vi "Istwerte eintragen.vi"(9 "Auswahlfelder":T1) -> (1 "Aktuelle Werte":T3 {"Zahlen-Ausgabefeld 16" format="%#.2f"; "Zahlen-Ausgabefeld 15" format="%#.2f"; "Zahlen-Ausgabefeld 14" format="%#.2f"; "Zahlen-Ausgabefeld 13" format="%#.2f"; "Zahlen-Ausgabefeld 12" format="%#.2f"; "Zahlen-Ausgabefeld 11" format="%#.2f"; "Zahlen-Ausgabefeld 10" format="%#.2f"; "Zahlen-Ausgabefeld 9" format="%#.2f"; "Zahlen-Ausgabefeld 8" format="%#.2f"; "Zahlen-Ausgabefeld 7" format="%#.2f"; "Zahlen-Ausgabefeld 6" format="%#.2f"; "Zahlen-Ausgabefeld 5" format="%#.2f"; "Zahlen-Ausgabefeld 4" format="%#.2f"; "Zahlen-Ausgabefeld 3" format="%#.2f"; "Zahlen-Ausgabefeld 2" format="%#.2f"; "Zahlen-Ausgabefeld" format="%#.2f"})   [LabVIEW 2020, in "Gaszuordnung AO.lvlib"]
uses:
  Gaszuordnung AO.lvlib
  Aktuelle Werte Anzeige.ctl
  Auswahlfelder Anzeige.ctl
  Visualisierungs Elemente/Auswahlfeld.ctl
  Messdaten/Messdaten.lvlib
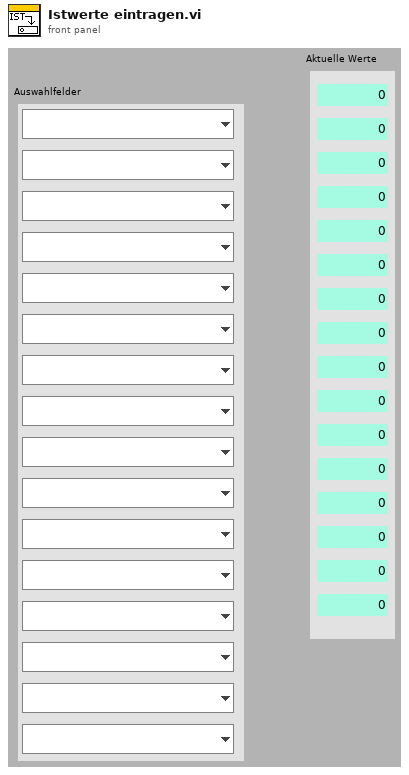
[diagram p1: front panel]
types:
  T1 = typedef "Gaszuordnung AO.lvlib/Auswahlfelder Anzeige.ctl" = cluster{"Auswahl":T2, "Auswahl 2":T2, "Auswahl 3":T2, "Auswahl 4":T2, "Auswahl 5":T2, "Auswahl 6":T2, "Auswahl 7":T2, "Auswahl 8":T2, "Auswahl 9":T2, "Auswahl 10":T2, "Auswahl 11":T2, "Auswahl 12":T2, "Auswahl 13":T2, "Auswahl 14":T2, "Auswahl 15":T2, "Auswahl 16":T2}
  T2 = typedef "Auswahlfeld.ctl" = u16
  T3 = typedef "Gaszuordnung AO.lvlib/Aktuelle Werte Anzeige.ctl" = cluster{"Zahlen-Ausgabefeld":sgl, "Zahlen-Ausgabefeld 2":sgl, "Zahlen-Ausgabefeld 3":sgl, "Zahlen-Ausgabefeld 4":sgl, "Zahlen-Ausgabefeld 5":sgl, "Zahlen-Ausgabefeld 6":sgl, "Zahlen-Ausgabefeld 7":sgl, "Zahlen-Ausgabefeld 8":sgl, "Zahlen-Ausgabefeld 9":sgl, "Zahlen-Ausgabefeld 10":sgl, "Zahlen-Ausgabefeld 11":sgl, "Zahlen-Ausgabefeld 12":sgl, "Zahlen-Ausgabefeld 13":sgl, "Zahlen-Ausgabefeld 14":sgl, "Zahlen-Ausgabefeld 15":sgl, "Zahlen-Ausgabefeld 16":sgl}
  T4 = cluster{"[0]":sgl, "[1]":sgl, "[2]":sgl, "[3]":sgl, "[4]":sgl, "[5]":sgl, "[6]":sgl, "[7]":sgl, "[8]":sgl, "[9]":sgl, "[10]":sgl, "[11]":sgl, "[12]":sgl, "[13]":sgl, "[14]":sgl, "[15]":sgl}
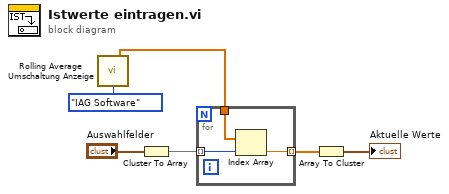
[diagram p0: block diagram]
diagram:
  n1 = call "Rolling Average Umschaltung Anzeige.vi"("Aktion"=enum16{"AK", "IAG Software"}."IAG Software") -> ("Aktuelle Messwerte"=w2:sgl[])  [unwired: 9 in, 5 out]
  n2 = Cluster To Array(cluster="Auswahlfelder") -> (array=w6:T2[])
  n3 = for {
    tunnel: w6 -> [w8] mode=indexing
    tunnel: w2 -> [w9]
    tunnel: [w7] -> w5 mode=indexing
    n4 = Index Array(array=w9, index=w8) -> (element=w7:sgl)
  }
  n5 = Array To Cluster(array=w5) -> (cluster=→"Aktuelle Werte":T4)
